vi "Get array of String.vi"(8 "error in (no error)":errorcluster, 11 "json class in":refnum<class "json class.lvclass">) -> (0 "error out":errorcluster, 2 "String Array":string[](array[string]), 3 "json class out":refnum<class "json class.lvclass">)   [LabVIEW 2021, in "Config Library.lvlib" / "json class.lvclass"]
uses:
  json class.lvclass
  json class.lvclass/json class.ctl
  <vilib>/addons/JSON API/JSON Value/JSON Value.lvclass
  <vilib>/addons/JSON API/JSON Scalar/JSON Scalar.lvclass
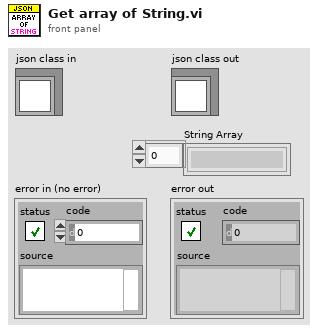
[diagram p1: front panel]
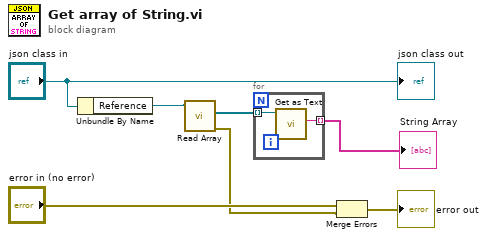
[diagram p0: block diagram]
diagram:
  n1 = Unbundle By Name("json class in") -> ("Reference"=w3:refnum<class "JSON Value.lvclass">)
  n2 = call-dynamic "Read Array.vi"("JSON Value In"=w3) -> ("error out"=w1:errorcluster, "Array"=w2:refnum<class "JSON Value.lvclass">[])  [unwired: 8 in, 1 out]
  n3 = for {
    tunnel: w2 -> [w9] mode=indexing
    tunnel: [w8] -> w4 mode=indexing
    n4 = call <vilib>:"Get as Text.vi"("JSON Scalar in"=w9) -> ("LabVIEW Text"=w8:string)  [unwired: 8 in, 2 out]
  }
  "String Array" <- w4
  n5 = Merge Errors("error in (no error)", w1) -> (→"error out":errorcluster)
  "json class out" <- "json class in"
